vi "Set_LJ_Port.vi"(8 "error in":errorcluster, 9 "State":bool=TRUE, 10 "Channel":enum16{"1", "2", "3", "4", "5", "6", "7", "8"}(ring), 11 "Flowboard":enum16{"A", "B", "C"}(ring)) -> (0 "error out":errorcluster)   [LabVIEW 2016]
uses:
  Globals/LJ_Handles_Global.vi
panel:
  out "Handle Out":i32
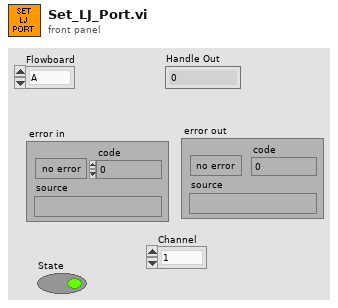
[diagram p1: front panel]
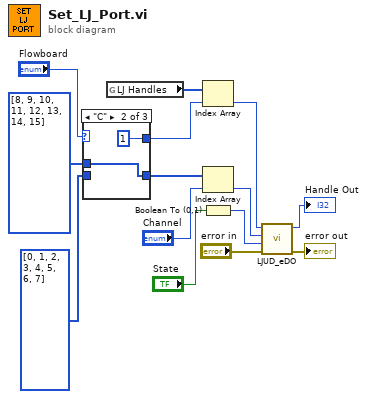
[diagram p0: block diagram]
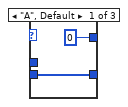
[diagram p2: hidden frame]
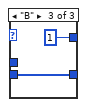
[diagram p3: hidden frame]
diagram:
  n1 = case shown="\"C\"" "Flowboard" {
    tunnel: [0 1 1] -> w6
    tunnel: i32[] [0, 1, 2, 3, 4, 5, 6, 7] ("LJ Handles") -> [w15 _ w19]
    tunnel: [w15 w17 w19] -> w3
    tunnel: i32[] [8, 9, 10, 11, 12, 13, 14, 15] ("LJ Handles") -> [_ w17 _]
    frame "A", Default {
    }
    frame "C" {
    }
    frame "B" {
    }
  }
  n2 = global read "LJ_Handles_Global.vi" "LJ Handles"() -> (w12:i32[])
  n3 = Index Array(array=w12, index=w6) -> (element=w11:i32)
  n4 = Index Array(array=w3, index="Channel") -> (element=w2:i32)
  n5 = Boolean To (0,1)(Boolean="State") -> (0, 1=w14:i16)
  n6 = call "LJUD_eDO.vi"("error in"="error in", "State"=w14, "Channel"=w2, "Handle In"=w11) -> ("error out"=→"error out":errorcluster, "Handle Out"=→"Handle Out":i32)  [unwired: 6 in]
